vi "CS++PreconfiguredContent.vi"() -> (0 "CS++Classes & Messages":T1(array[cluster]))   [LabVIEW 2016]
doc: "Place actor and class constants that should be included included in an application on the blockdiagramm."
uses:
  <vilib>/ActorFramework/Message/Message.lvclass
  CSPP_DIM/Examples/CS++DIM-Client/CS++DIM-Client.lvclass
  CSPP_DIM/Examples/CS++DIM-Server/CS++DIM-Server.lvclass
  CSPP_Syslog/CS++Syslog.lvclass
  Actors/CS++BaseActor/CS++BaseActor.lvclass
panel:
  # "Place actor and class constants on the blockdiagramm."
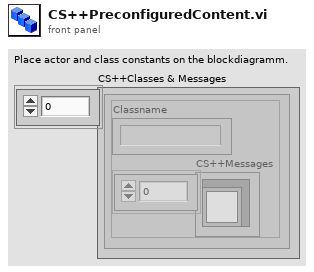
[diagram p1: front panel]
types:
  T1 = cluster{"Classname":string, "CS++Messages":refnum<class "Message.lvclass">[]}[]
  T2 = cluster{"class name":string, "CS++Messages":refnum<class "Message.lvclass">[]}
  T3 = cluster{"class name":string, "CS++Messages":refnum<class "Message.lvclass">[]}[]
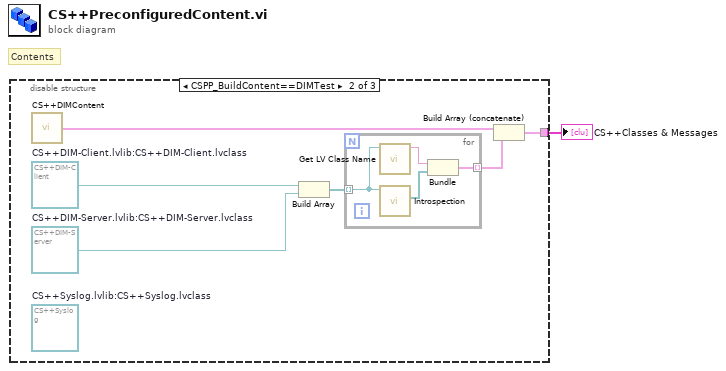
[diagram p0: block diagram]
diagram:
  # "Contents"
  n1 = disable-structure shown="CSPP_BuildContent==DIMTest" {
    disable-tunnel: [_ w2 _] -> w1
    frame condition #0 (active) {
    }
    frame condition #1 {
      (unwired) refnum<class "CS++Syslog.lvclass"> refnum  # CS++Syslog.lvlib:CS++Syslog.lvclass
      w6 = refnum<class "CS++DIM-Server.lvclass"> refnum  # CS++DIM-Server.lvlib:CS++DIM-Server.lvclass
      w7 = refnum<class "CS++DIM-Client.lvclass"> refnum  # CS++DIM-Client.lvlib:CS++DIM-Client.lvclass
      n2 = call "CS++DIMContent.vi"() -> ("CS++Classes & Messages"=w4:T1)  [unwired: 1 in]
      n3 = Build Array(w7, w6) -> (w5:refnum<class>[])
      n4 = for {
        tunnel: w5 -> [w11] mode=indexing
        tunnel: [w8] -> w3 mode=indexing
        n5 = call <vilib>:"Get LV Class Name.vi"("object"=w11) -> ("class name"=w10:string)  [unwired: 9 in, 1 out]
        n6 = call "Introspection.vi"("CS++BaseActor in"=w11) -> ("CS++Messages"=w9:refnum<class "Message.lvclass">[])  [unwired: 8 in, 2 out]
        n7 = Bundle("class name"=w10, "CS++Messages"=w9) -> (w8:T2)  [unwired: 1 in]
      }
      n8 = Build Array (concatenate)(w4, w3) -> (w2:T3)
    }
    frame condition #2 {
    }
  }
  "CS++Classes & Messages" <- w1
